vi "ReadUDP.vi"(3 "error in (no error)":errorcluster, 4 "connection ID":refnum<k16>, 5 "Message length":u16=10) -> (0 "error out":errorcluster, 1 "Discarding":bool, 2 "Array":u8[][](array[numeric])=[[2, 225, 14, 196, 12, 0, 0, 0, 0, 0], [2, 226, 35, 253, 12, 0, 0, 0, 0, 0], [2, 227, 56, 248, 12, 0, 0, 0, 0, 0], [2, 228, 77, 195, 12, 0, 0, 0, 0, 0], [2, 241, 7, 28, 0, 0, 0, 0, 0, 0], [2, 242, 14, 27, 0, 0, 0, 0, 0, 0], [2, 243, 21, 29, 0, 0, 0, 0, 0, 0], [2, 244, 28, 28, 0, 0, 0, 0, 0, 0], [0, 144, 12, 42, 12, 247, 12, 20, 12, 129], [0, 112, 11, 37, 0, 225, 1, 0, 0, 0], [0, 113, 15, 104, 8, 4, 1, 0, 0, 0], [2, 0, 2, 4, 5, 5, 2, 0, 0, 0], [0, 98, 3, 242, 1, 24, 0, 131, 0, 0], [0, 99, 46, 33, 1, 1, 1, 1, 1, 44], [0, 102, 2, 71, 1, 51, 0, 74, 0, 0], [0, 103, 33, 35, 1, 1, 1, 1, 1, 44]])   [LabVIEW 2017]
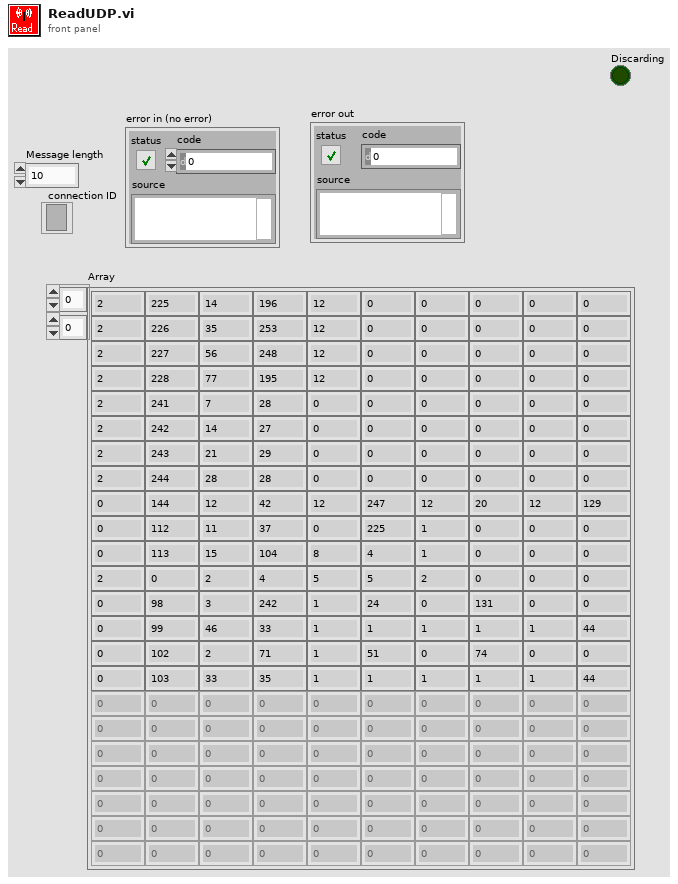
[diagram p1: front panel]
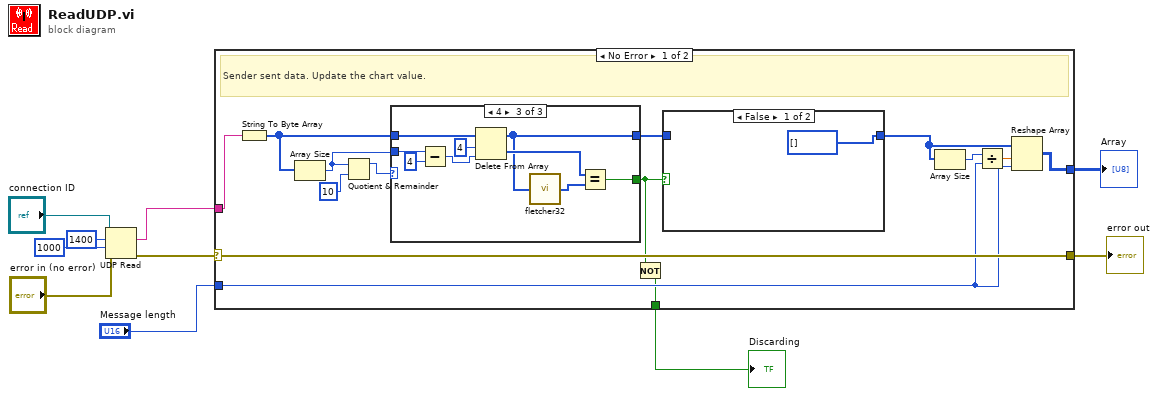
[diagram p0: block diagram]
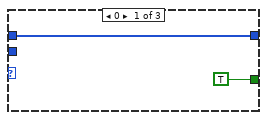
[diagram p3: hidden frame]
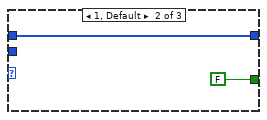
[diagram p4: hidden frame]
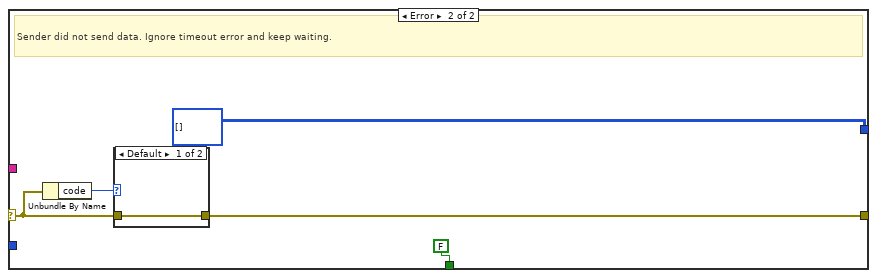
[diagram p5: hidden frame]
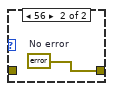
[diagram p6: hidden frame]
diagram:
  n1 = UDP Read(connection ID="connection ID", max size (548)=1400, timeout ms (25000)=1000, 8:"error in (no error)") -> (data out=w8:string, error out=w2:errorcluster)  [unwired: 3 out]
  n2 = case shown="No Error" w2 {
    selector: w2 -> [w24 w43]
    tunnel: w8 -> [w23 _]
    tunnel: [w24 w42] -> w3
    tunnel: [w20 u8[][] [] ("unsigned byte array")] -> w7
    tunnel: "Message length" -> [w19 _]
    tunnel: [w11 FALSE] -> w1
    frame No Error {
      # "Sender sent data. Update the chart value."
      n3 = String To Byte Array(string=w23) -> (unsigned byte array=w18:u8[])
      n4 = Array Size(array=w18) -> (size(s)=w16:i32)
      n5 = Quotient & Remainder(x=w16, y=10) -> (x-y*floor(x/y)=w15:i32)  [unwired: 1 out]
      n6 = case shown="4" w15 {
        tunnel: w18 -> [w28 w30 w39]
        tunnel: [w28 w30 w32] -> w14
        tunnel: w16 -> [_ _ w37]
        tunnel: [TRUE FALSE w31] -> w12
        frame 0 {
        }
        frame 1, Default {
        }
        frame 4 {
          n7 = Subtract(x=w37, y=4) -> (x-y=w35:i32)
          n8 = Delete From Array(array=w39, length=4, index=w35) -> (deleted portion=w34:u8[], array with subset deleted=w32:u8[])
          n9 = call "fletcher32.vi"("UPDread out"=w32) -> ("checksum"=w33:u8[])
          n10 = Equal?(x=w34, y=w33) -> (x = y?=w31:bool)
        }
      }
      n11 = Not(x=w12) -> (.not. x?=w11:bool)
      n12 = case shown="False" w12 {
        tunnel: w14 -> [_ w26]
        tunnel: [u8[] [] ("unsigned byte array") w26] -> w13
        frame False {
        }
        frame True {
        }
      }
      n13 = Array Size(array=w13) -> (size(s)=w22:i32)
      n14 = Divide(x=w22, y=w19) -> (x/y=w21:dbl)
      n15 = Reshape Array(w13, w21, w19) -> (w20:u8[][])
    }
    frame Error {
      # "Sender did not send data. Ignore timeout error and keep waiting."
      n16 = Unbundle By Name(w43) -> ("code"=w44:i32)
      n17 = case shown="Default" w44 {
        tunnel: w43 -> [w45 _]
        tunnel: [w45 w46] -> w42
        frame Default {
        }
        frame 56 {
          w46 = errorcluster {"status"=FALSE, "code"=0, "source"=""}  # No error
        }
      }
    }
  }
  "Array" <- w7
  "error out" <- w3
  "Discarding" <- w1
